vi "historico_calibraçcao.vi"() -> ()   [LabVIEW 2016]
panel:
  out "Histórico":dbl[][](array[numeric])
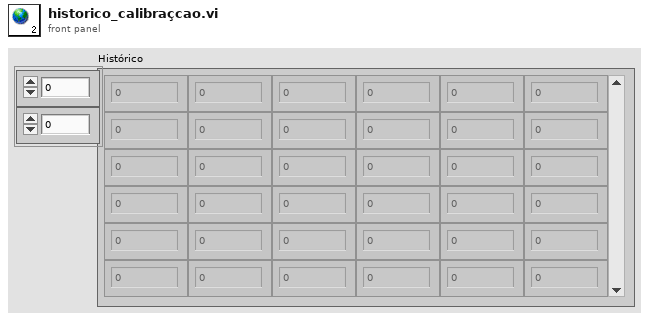
[diagram p1: front panel]
diagram:
